vi "Word_Insert_Line.vi"(0 "Word.InlineShapes":refnum<k7>, 1 "size (default)":i32, 2 "noshade (F)":bool, 5 "Word._Document":refnum<k7>, 7 "align (default)":enum16{"(default)", "LEFT", "CENTER", "RIGHT"}(ring), 9 "bookmark (Word)":string, 11 "error in":errorcluster, 12 "Insertion point":u16, 13 "width (0=default)":dbl format="%.2f", 14 "width units":enum16{"Pixels", "Percentage"}(ring)) -> (15 "error out":errorcluster)   [LabVIEW 2017, in "NI_ReportGenerationToolkit.lvlib"]
uses:
  <vilib>/addons/_office/NI_ReportGenerationToolkit.lvlib
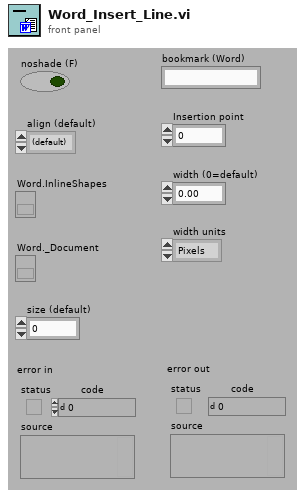
[diagram p1: front panel]
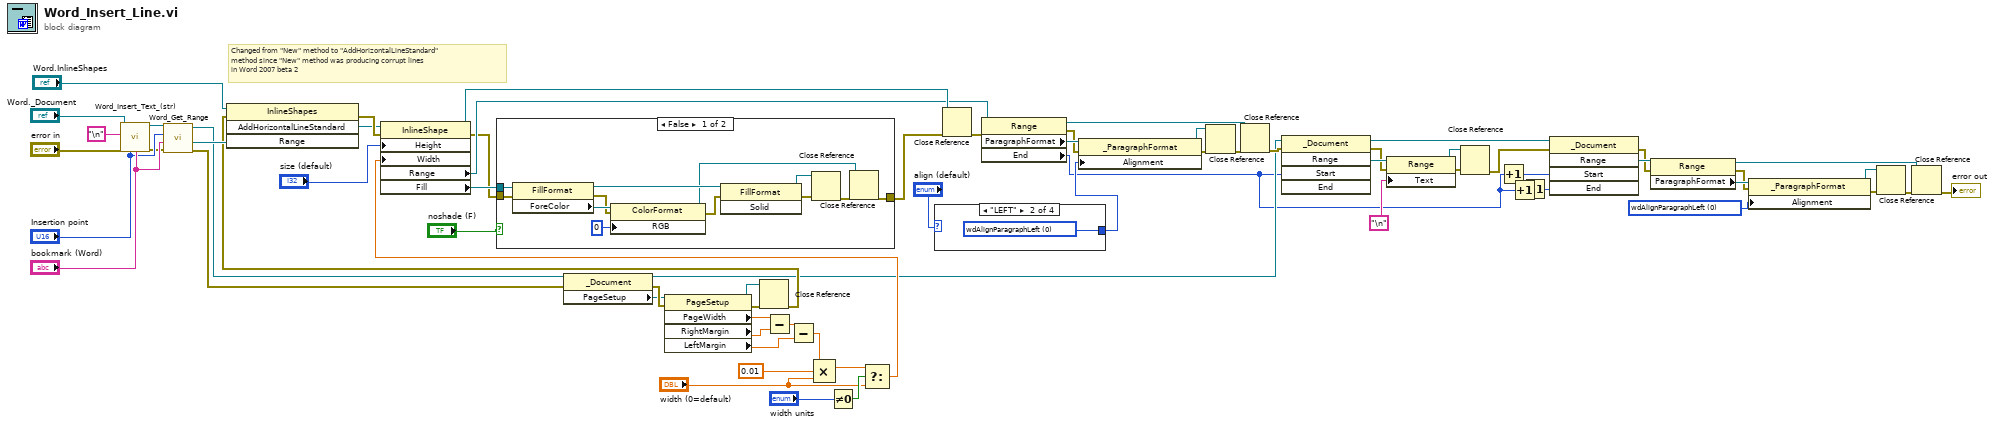
[diagram p0: block diagram]
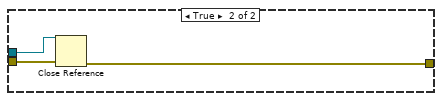
[diagram p2: hidden frame]
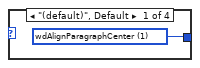
[diagram p3: hidden frame]
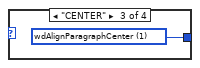
[diagram p4: hidden frame]
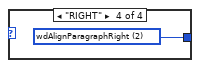
[diagram p5: hidden frame]
diagram:
  w22 = 0 items=["wdAlignParagraphLeft", "wdAlignParagraphCenter", "wdAlignParagraphRight", "wdAlignParagraphJustify"] ("Alignment")
  # "Changed from \"New\" method to \"AddHorizontalLineStandard\"\nmethod since \"New\" method was producing corrupt lines\nin Word 2007 beta 2"
  n1 = call <vilib>:"Word_Insert_Text_(str).vi"("Word._Document"="Word._Document", "Text"="\n", "Error in (no error)"="error in", "Insertion point"="Insertion point", "Bookmark name"="bookmark (Word)") -> ("ActiveDocument out"=w65:refnum<k7>, "Error out"=w63:errorcluster)  [unwired: 5 in, 4 out]
  n2 = call <vilib>:"Word_Get_Range.vi"("error in"=w63, "bookmark name"="bookmark (Word)", "insertion point"="Insertion point", "document in"=w65) -> ("error out (no error)"=w60:errorcluster, "range"=w61:refnum<k7>, "document out"=w59:refnum<k7>)  [unwired: 2 in, 3 out]
  n3 = property class="_Document"(reference=w59, error in=w60) -> (reference out=w15:refnum<k7>, error out=w53:errorcluster, "PageSetup"=w46:refnum<k7>)
  n4 = property class="PageSetup"(reference=w46, error in=w53) -> (reference out=w58:refnum<k7>, error out=w54:errorcluster, "PageWidth"=w43:sgl, "RightMargin"=w42:sgl, "LeftMargin"=w40:sgl)
  n5 = Close Reference(reference=w58, error in (no error)=w54) -> (error out=w55:errorcluster)
  n6 = invoke class="InlineShapes" method="AddHorizontalLineStandard"(reference="Word.InlineShapes", error in=w55, "Range"=w61) -> (error out=w56:errorcluster, "AddHorizontalLineStandard"=w38:refnum<k7>)  [unwired: 1 in, 2 out]
  n7 = Subtract(x=w43, y=w42) -> (x-y=w41:sgl)
  n8 = Subtract(x=w41, y=w40) -> (x-y=w39:sgl)
  n9 = Compound Arithmetic op=MULTIPLY(w39, 0.01, "width (0=default)") -> (w48:dbl)
  n10 = Not Equal To 0?(x="width units") -> (x != 0?=w51:bool)
  n11 = Select(t=w48, s=w51, f="width (0=default)") -> (s? t:f=w52:dbl)
  n12 = property class="InlineShape"(reference=w38, error in=w56, "Height"="size (default)", "Width"=w52) -> (reference out=w57:refnum<k7>, error out=w2:errorcluster, "Range"=w37:refnum<k7>, "Fill"=w4:refnum<k7>)
  n13 = case shown="False" "noshade (F)" {
    tunnel: w4 -> [w80 w82]
    tunnel: w2 -> [w74 w83]
    tunnel: [w71 w81] -> w1
    frame False {
      n14 = property class="FillFormat"(reference=w80, error in=w74) -> (reference out=w76:refnum<k7>, error out=w78:errorcluster, "ForeColor"=w79:refnum<k7>)
      n15 = property class="ColorFormat"(reference=w79, error in=w78, "RGB"=0) -> (reference out=w69:refnum<k7>, error out=w75:errorcluster)
      n16 = invoke class="FillFormat" method="Solid"(reference=w76, error in=w75) -> (reference out=w70:refnum<k7>, error out=w73:errorcluster)  [unwired: 1 in, 1 out]
      n17 = Close Reference(reference=w70, error in (no error)=w73) -> (error out=w72:errorcluster)
      n18 = Close Reference(reference=w69, error in (no error)=w72) -> (error out=w71:errorcluster)
    }
    frame True {
      n19 = Close Reference(reference=w82, error in (no error)=w83) -> (error out=w81:errorcluster)
    }
  }
  n20 = case shown="\"LEFT\"" "align (default)" {
    tunnel: [w84 w85 w86 w87] -> w28
    frame "(default)", Default {
      w84 = 1 items=["wdAlignParagraphLeft", "wdAlignParagraphCenter", "wdAlignParagraphRight", "wdAlignParagraphJustify"] ("Alignment")
    }
    frame "LEFT" {
      w85 = 0 items=["wdAlignParagraphLeft", "wdAlignParagraphCenter", "wdAlignParagraphRight", "wdAlignParagraphJustify"] ("Alignment")
    }
    frame "CENTER" {
      w86 = 1 items=["wdAlignParagraphLeft", "wdAlignParagraphCenter", "wdAlignParagraphRight", "wdAlignParagraphJustify"] ("Alignment")
    }
    frame "RIGHT" {
      w87 = 2 items=["wdAlignParagraphLeft", "wdAlignParagraphCenter", "wdAlignParagraphRight", "wdAlignParagraphJustify"] ("Alignment")
    }
  }
  n21 = Close Reference(reference=w57, error in (no error)=w1) -> (error out=w35:errorcluster)
  n22 = property class="Range"(reference=w37, error in=w35) -> (reference out=w30:refnum<k7>, error out=w34:errorcluster, "ParagraphFormat"=w36:refnum<k7>, "End"=w8:i32)
  n23 = property class="_ParagraphFormat"(reference=w36, error in=w34, "Alignment"=w28) -> (reference out=w31:refnum<k7>, error out=w33:errorcluster)
  n24 = Close Reference(reference=w31, error in (no error)=w33) -> (error out=w32:errorcluster)
  n25 = Close Reference(reference=w30, error in (no error)=w32) -> (error out=w27:errorcluster)
  n26 = invoke class="_Document" method="Range"(reference=w15, error in=w27, "Start"=w8) -> (reference out=w14:refnum<k7>, error out=w24:errorcluster, "Range"=w26:refnum<k7>)  [unwired: 2 in, 2 out]
  n27 = property class="Range"(reference=w26, error in=w24, "Text"="\n") -> (reference out=w12:refnum<k7>, error out=w13:errorcluster)
  n28 = Close Reference(reference=w12, error in (no error)=w13) -> (error out=w11:errorcluster)
  n29 = Increment(x=w8) -> (x+1=w6:i32)
  n30 = Increment(x=w8) -> (x+1=w7:i32)
  n31 = Increment(x=w7) -> (x+1=w5:i32)
  n32 = invoke class="_Document" method="Range"(reference=w14, error in=w11, "Start"=w6, "End"=w5) -> (error out=w9:errorcluster, "Range"=w10:refnum<k7>)  [unwired: 1 in, 3 out]
  n33 = property class="Range"(reference=w10, error in=w9) -> (reference out=w17:refnum<k7>, error out=w21:errorcluster, "ParagraphFormat"=w23:refnum<k7>)
  n34 = property class="_ParagraphFormat"(reference=w23, error in=w21, "Alignment"=w22) -> (reference out=w18:refnum<k7>, error out=w20:errorcluster)
  n35 = Close Reference(reference=w18, error in (no error)=w20) -> (error out=w19:errorcluster)
  n36 = Close Reference(reference=w17, error in (no error)=w19) -> (error out=→"error out":errorcluster)
